vi "MainRT.vi"() -> ()   [LabVIEW 2017]
doc: "Test \"RubikStartup.vi\".\n\nPut servos and gripps into start state (0° and closed).\nWaits 3sec so that you can position the cube.\nYou have to hold the cube at a correct position so that grippers can grab it.\nAfter 3sec grippers opens at vi stops."
uses:
  <vilib>/myRIO/Common/Instrument Driver Framework/myRIO v1.0/UART/vis/myRIO v1.0 Close UART.vi
  <vilib>/myRIO/Common/Instrument Driver Framework/Utilities/vis/FPGA Ref Manager.vi
  <vilib>/myRIO/Common/Instrument Driver Framework/myRIO v1.0/myRIO v1.0 Reset FPGA.vi
  <vilib>/myRIO/Common/Instrument Driver Framework/myRIO v1.0/IRQ/vis/myRIO v1.0 IRQ Info FGV.vi
  <vilib>/myRIO/Common/Instrument Driver Framework/myRIO v1.0/IRQ/vis/myRIO v1.0 Timer IRQ Info FGV.vi
  <vilib>/myRIO/Common/Instrument Driver Framework/myRIO v1.0/IRQ/vis/myRIO v1.0 ISR Agent.vi
  Projekt-RubikLibrary/RubikLibraryRT.lvlib
  <vilib>/myRIO/Instrument Drivers/Utilities/Utilities.lvlib
panel:
  out "Error Output":errorcluster
  # "Test Rubik's Cube Start Up"
  # "Turn all servos to 0°\nCloses all grippers and opens grippers after 9sec."
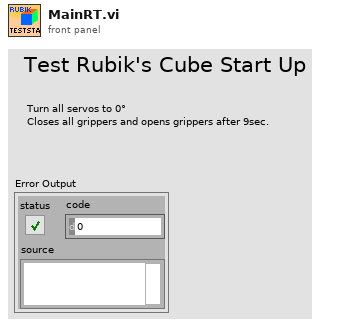
[diagram p1: front panel]
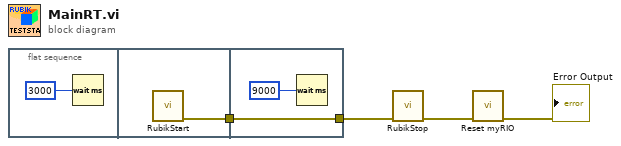
[diagram p0: block diagram]
diagram:
  n1 = flat-sequence {
    tunnel: [w6] -> w2
    tunnel: [w8] -> w1
    tunnel: w2 -> [w8]
    frame #0 {
      n2 = Wait (ms)(milliseconds to wait=u32 3000) -> ()  [unwired: 1 out]
    }
    frame #1 {
      n3 = call "RubikStart.vi"() -> ("error out"=w6:errorcluster)  [unwired: 11 in]
    }
    frame #2 {
      n4 = Wait (ms)(milliseconds to wait=u32 9000) -> ()  [unwired: 1 out]
    }
  }
  n5 = call "RubikStop.vi"("error in"=w1) -> ("error out"=w3:errorcluster)  [unwired: 10 in]
  n6 = call <vilib>:"Reset myRIO.vi"("error in (no error)"=w3) -> ("error out"=→"Error Output":errorcluster)  [unwired: 10 in]
